vi "Unpack Message.vi"(8 "error in (no error)":errorcluster, 9 "Packed Message":string, 10 "Message Name":string, 11 "Car Position Changed in":refnum<class "Car Position Changed.lvclass">) -> (0 "error out":errorcluster, 2 "Valid":bool, 3 "Car Position Changed out":refnum<class "Car Position Changed.lvclass">)   [LabVIEW 2016, in "CLD Exam - Car Wash.lvlib" / "Car Position Changed.lvclass"]
uses:
  Car Position Changed.lvclass
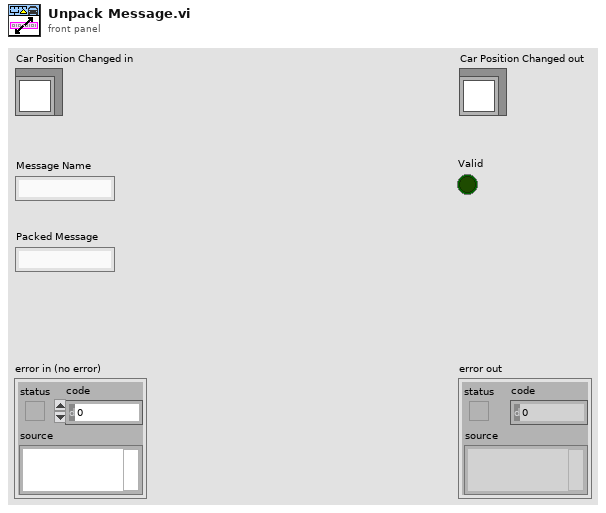
[diagram p1: front panel]
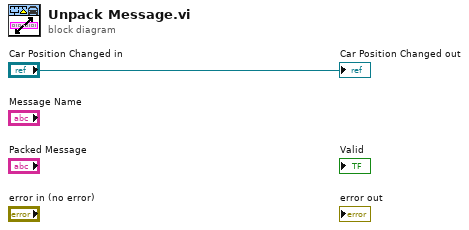
[diagram p0: block diagram]
diagram:
  "Car Position Changed out" <- "Car Position Changed in"
